vi "RT oscilloscope.vi"() -> ()   [LabVIEW 2023]
uses:
  <resource>/objmgr/ni.dex.rc
  <vilib>/rvi/interface/nirviReadWriteControl/nirviReadWriteControl.xnode
  <vilib>/rvi/interface/Simulation/niFpgaSimulationCallBeginRW.vi
  <vilib>/rvi/errors/niLvFpgaAdjustHostInterfaceError.vi
  <vilib>/rvi/interface/nirviMethod/nirviMethod.xnode
  <vilib>/FPGAPlugInAG/Dynamic/niLvFpga_Run_Dynamic.vi
  <vilib>/FPGAPlugInAG/Dynamic/niLvFpga_Reset_Dynamic.vi
  <vilib>/rvi/interface/nirviMethod/StockFPGA_InlinedMethodWaitForSingleIRQ.vi
  <vilib>/FPGAPlugInAG/Dynamic/niLvFpga_WaitOnIrq_Dynamic.vi
  <vilib>/FPGAPlugInAG/Dynamic/niLvFpga_AcknowledgeIrq_Dynamic.vi
  <vilib>/FPGAPlugInAG/Dynamic/niLvFpga_ReadFifo_Dynamic.vi
  <vilib>/rvi/errors/niLvFpgaMergeErrorWithErrorCode.vi
  <vilib>/rvi/interface/nirviOpenFPGA/nirviOpenFPGA.xnode
  <vilib>/rvi/interface/nirviCloseFPGA/nirviCloseFPGA.xnode
  <vilib>/FPGAPlugInAG/Dynamic/niLvFpga_Close_Dynamic.vi
  FPGA Bitfiles/Mainproject_FPGATarget_Icreadoutclocked_PcJtOPDfEmI.lvbitx
  Ic readout_clocked_delayed trigger_dist V3.vi
  Transport measurement/FPGA Bitfiles/transportmain_FPGATarget_oscilloscope_quBCWYi9ZeU.lvbitx
  oscilloscope.vi
  <vilib>/FPGAPlugInAG/cRIO-9063/niLvFpga_Open_cRIO-9063.vi
  <vilib>/rvi/interface/common/dynamic/niFpgaDynamicAddResources.vi
  <vilib>/LabVIEW Targets/FPGA/cRIO/shared/nicrio_ModuleControls/nicrio_cRIO-9775_RecordDataRates4ChansRing.ctl
  RT fast data.ctl
panel:
  out "VI Stop":bool
  out "error out 2":errorcluster
  out "error out":errorcluster
  in  "Parameters":T1={"Records Num"=10000, "AI Trigger Configuration"={"Trigger Slope"=enum."Positive", "Trigger Level"=0.1298828125, "Hystesis Value"=0.0, "AI Channel"=0}, "Record PreTrigger Samples"=1, "Record Samples"=16, "Ic Cut off or curve"=TRUE, "Gate wait time us"=150, "Record Data Rate"=1, "Count us half of T"=15, "Wait before trigger us"=10100, "Cutoff delay usec"=0} {"Record Data Rate" items=["20.000 MS/s (NI 9775)"=1, "10.00 MS/s (NI 9775)"=2, "6.667 MS/s (NI 9775)"=3, "5.000 MS/s (NI 9775)"=4, "2.500 MS/s (NI 9775)"=8, "1.667 MS/s (NI 9775)"=12, "1.250 MS/s (NI 9775)"=16, "1.000 MS/s (NI 9775)"=20, "833.333 KS/s (NI 9775)"=24, "714.286 KS/s (NI 9775)"=28, "625.000 KS/s (NI 9775)"=32, "555.556 KS/s (NI 9775)"=36, "500.000 KS/s (NI 9775)"=40, "454.545 KS/s (NI 9775)"=44, "416.667 KS/s (NI 9775)"=48, "384.615 KS/s (NI 9775)"=52, "357.143 KS/s (NI 9775)"=56, "333.333 KS/s (NI 9775)"=60, "312.500 KS/s (NI 9775)"=64, "294.118 KS/s (NI 9775)"=68, "277.778 KS/s (NI 9775)"=72, "263.158 KS/s (NI 9775)"=76, "250.000 KS/s (NI 9775)"=80, "238.095 KS/s (NI 9775)"=84, "227.273 KS/s (NI 9775)"=88, "217.391 KS/s (NI 9775)"=92, "208.333 KS/s (NI 9775)"=96, "200.000 KS/s (NI 9775)"=100, "192.308 KS/s (NI 9775)"=104, "185.185 KS/s (NI 9775)"=108, "178.571 KS/s (NI 9775)"=112, "172.414 KS/s (NI 9775)"=116, "166.667 KS/s (NI 9775)"=120, "161.290 KS/s (NI 9775)"=124, "156.250 KS/s (NI 9775)"=128, "151.515 KS/s (NI 9775)"=132, "147.059 KS/s (NI 9775)"=136, "142.857 KS/s (NI 9775)"=140, "138.889 KS/s (NI 9775)"=144, "135.135 KS/s (NI 9775)"=148, "131.579 KS/s (NI 9775)"=152, "128.205 KS/s (NI 9775)"=156, "125.000 KS/s (NI 9775)"=160, "121.951 KS/s (NI 9775)"=164, "119.048 KS/s (NI 9775)"=168, "116.279 KS/s (NI 9775)"=172, "113.636 KS/s (NI 9775)"=176, "111.111 KS/s (NI 9775)"=180, "108.696 KS/s (NI 9775)"=184, "106.383 KS/s (NI 9775)"=188, "104.167 KS/s (NI 9775)"=192, "102.041 KS/s (NI 9775)"=196, "100.000 KS/s (NI 9775)"=200, "50.000 KS/s (NI 9775)"=400, "33.333 KS/s (NI 9775)"=600, "25.000 KS/s (NI 9775)"=800, "20.000 KS/s (NI 9775)"=1000, "16.667 KS/s (NI 9775)"=1200, "14.286 KS/s (NI 9775)"=1400, "12.500 KS/s (NI 9775)"=1600, "11.111 KS/s (NI 9775)"=1800, "10.000 KS/s (NI 9775)"=2000, "9.091 KS/s (NI 9775)"=2200, "8.333 KS/s (NI 9775)"=2400, "7.692 KS/s (NI 9775)"=2600, "7.143 KS/s (NI 9775)"=2800, "6.667 KS/s (NI 9775)"=3000, "6.250 KS/s (NI 9775)"=3200, "5.882 KS/s (NI 9775)"=3400, "5.556 KS/s (NI 9775)"=3600, "5.000 KS/s (NI 9775)"=4000, "4.762 KS/s (NI 9775)"=4200, "4.545 KS/s (NI 9775)"=4400, "4.348 KS/s (NI 9775)"=4600, "4.167 KS/s (NI 9775)"=4800, "4.000 KS/s (NI 9775)"=5000, "3.846 KS/s (NI 9775)"=5200, "3.571 KS/s (NI 9775)"=5600, "3.333 KS/s (NI 9775)"=6000, "3.125 KS/s (NI 9775)"=6400, "2.941 KS/s (NI 9775)"=6800, "2.778 KS/s (NI 9775)"=7200, "2.632 KS/s (NI 9775)"=7600, "2.500 KS/s (NI 9775)"=8000, "2.381 KS/s (NI 9775)"=8400, "2.273 KS/s (NI 9775)"=8800, "2.174 KS/s (NI 9775)"=9200, "2.083 KS/s (NI 9775)"=9600, "2.000 KS/s (NI 9775)"=10000, "1.923 KS/s (NI 9775)"=10400, "1.852 KS/s (NI 9775)"=10800, "1.786 KS/s (NI 9775)"=11200, "1.724 KS/s (NI 9775)"=11600, "1.667 KS/s (NI 9775)"=12000, "1.613 KS/s (NI 9775)"=12400, "1.563 KS/s (NI 9775)"=12800, "1.515 KS/s (NI 9775)"=13200, "1.471 KS/s (NI 9775)"=13600, "1.429 KS/s (NI 9775)"=14000, "1.389 KS/s (NI 9775)"=14400, "1.351 KS/s (NI 9775)"=14800, "1.316 KS/s (NI 9775)"=15200, "1.282 KS/s (NI 9775)"=15600, "1.250 KS/s (NI 9775)"=16000, "1.220 KS/s (NI 9775)"=16400, "1.190 KS/s (NI 9775)"=16800, "1.163 KS/s (NI 9775)"=17200, "1.136 KS/s (NI 9775)"=17600, "1.111 KS/s (NI 9775)"=18000, "1.087 KS/s (NI 9775)"=18400, "1.064 KS/s (NI 9775)"=18800, "1.042 KS/s (NI 9775)"=19200, "1.020 KS/s (NI 9775)"=19600, "1.000 KS/s (NI 9775)"=20000, "0.980 KS/s (NI 9775)"=20400, "0.962 KS/s (NI 9775)"=20800, "0.943 KS/s (NI 9775)"=21200, "0.926 KS/s (NI 9775)"=21600, "0.909 KS/s (NI 9775)"=22000, "0.893 KS/s (NI 9775)"=22400, "0.877 KS/s (NI 9775)"=22800, "0.862 KS/s (NI 9775)"=23200, "0.847 KS/s (NI 9775)"=23600, "0.833 KS/s (NI 9775)"=24000, "0.820 KS/s (NI 9775)"=24400, "0.806 KS/s (NI 9775)"=24800, "0.794 KS/s (NI 9775)"=25200, "0.781 KS/s (NI 9775)"=25600, "0.694 KS/s (NI 9775)"=28800, "0.625 KS/s (NI 9775)"=32000, "0.568 KS/s (NI 9775)"=35200, "0.521 KS/s (NI 9775)"=38400, "0.446 KS/s (NI 9775)"=44800, "0.391 KS/s (NI 9775)"=51200, "0.347 KS/s (NI 9775)"=57600, "0.313 KS/s (NI 9775)"=64000]}
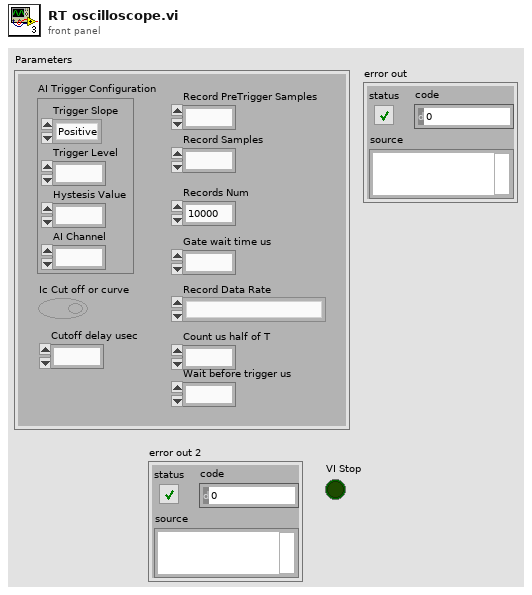
[diagram p1: front panel]
types:
  T1 = typedef "RT fast data.ctl" = cluster{"Records Num":i32, "AI Trigger Configuration":cluster{"Trigger Slope":enum8{"Positive", "Negative"}, "Trigger Level":fxp<+/-,17,5>, "Hystesis Value":fxp<+,16,4>, "AI Channel":u8}, "Record PreTrigger Samples":u32, "Record Samples":u32, "Ic Cut off or curve":bool, "Gate wait time us":u32, "Record Data Rate":T2, "Count us half of T":u32, "Wait before trigger us":u32, "Cutoff delay usec":u32}
  T2 = typedef "nicrio_cRIO-9775_RecordDataRates4ChansRing.ctl" = u16
  T3 = cluster{"Command":string, "Voltage":dbl, "Channel":string}
  T4 = cluster{"Trigger Slope":enum8{"Positive", "Negative"}, "Trigger Level":fxp<+/-,17,5>, "Hystesis Value":fxp<+,16,4>, "AI Channel":u8}
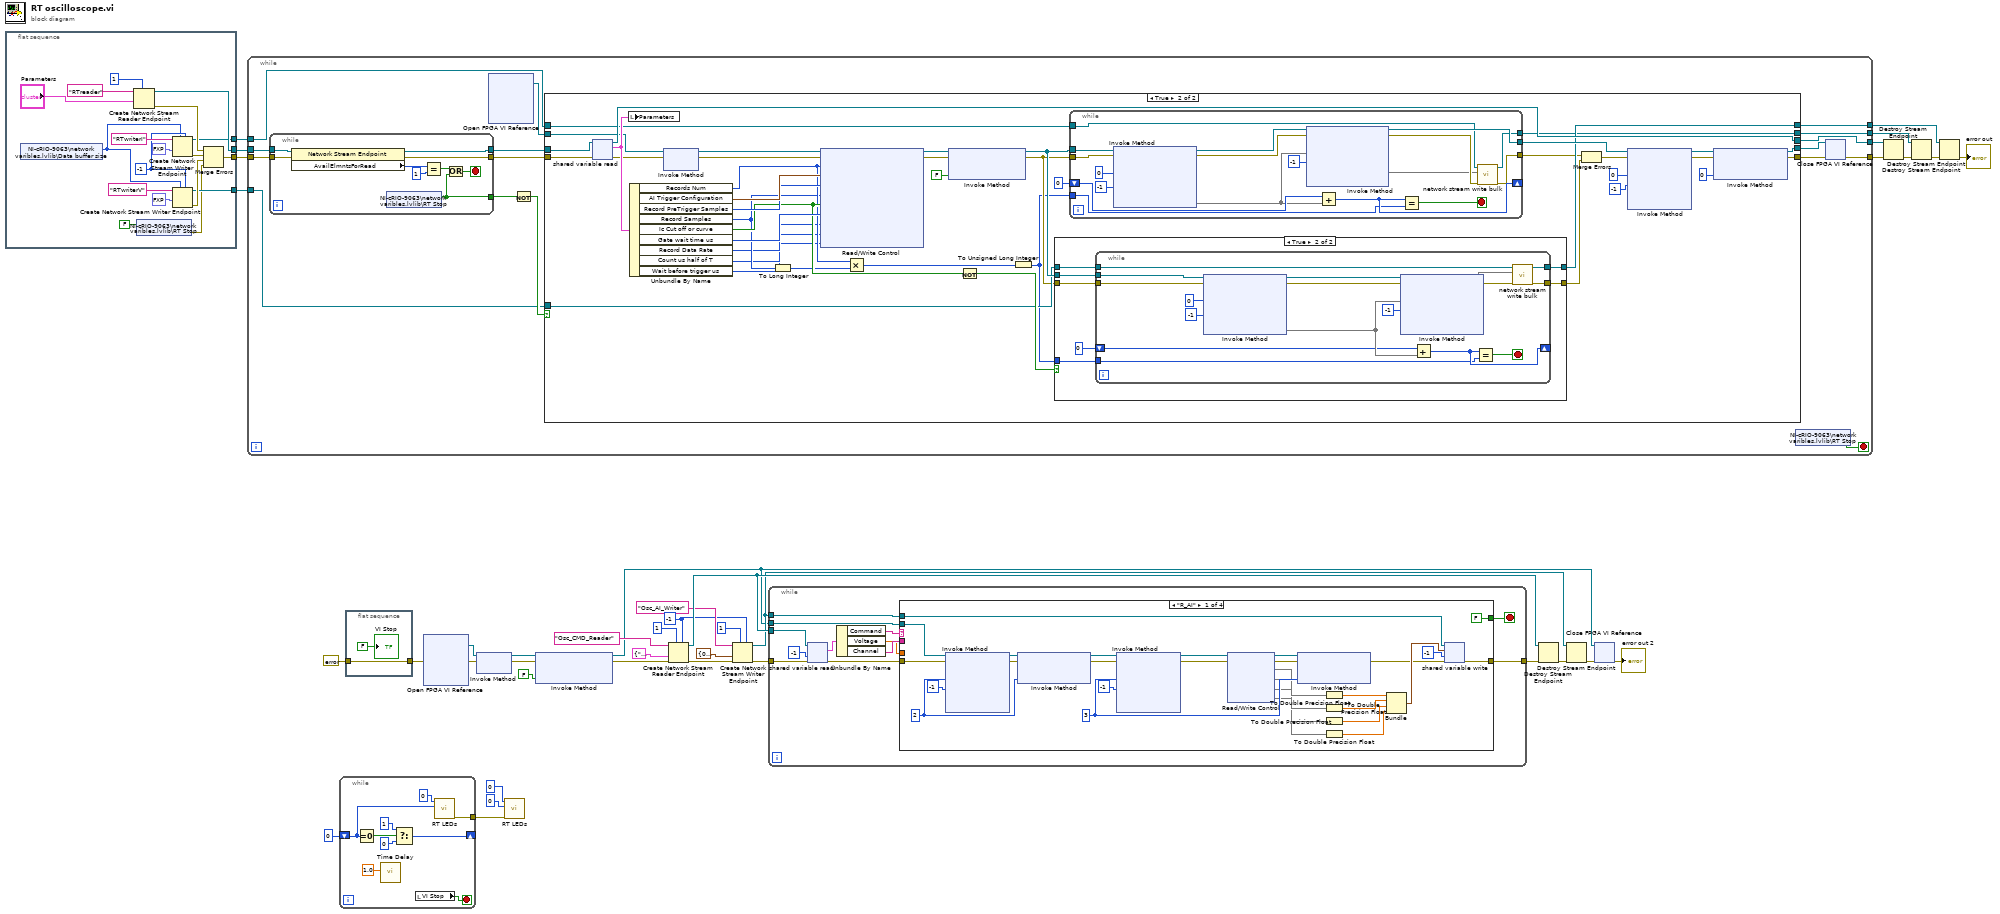
[diagram p0: block diagram]
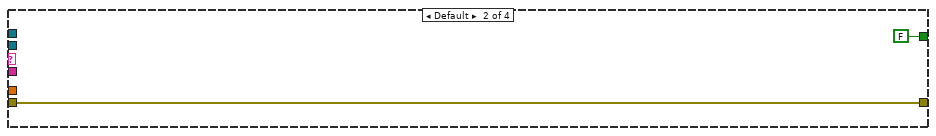
[diagram p2: hidden frame]
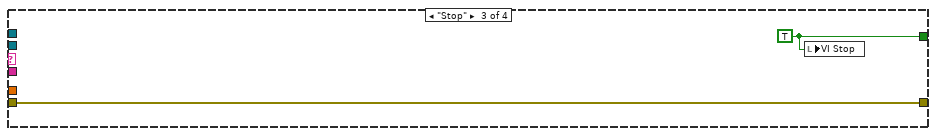
[diagram p3: hidden frame]
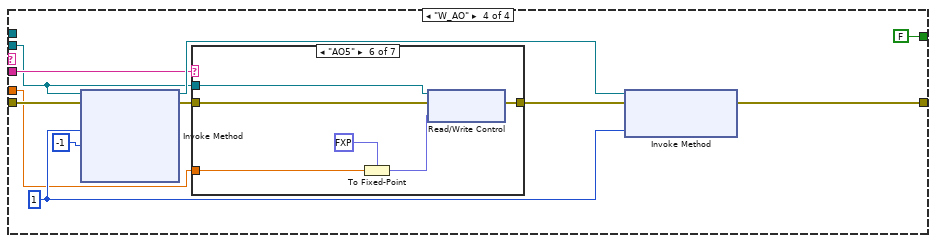
[diagram p4: hidden frame]
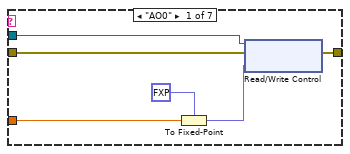
[diagram p5: hidden frame]
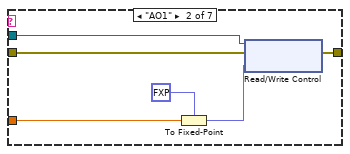
[diagram p6: hidden frame]
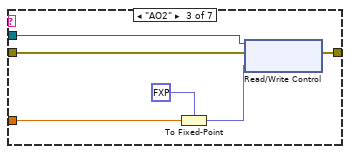
[diagram p7: hidden frame]
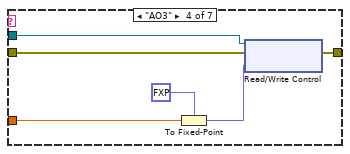
[diagram p8: hidden frame]
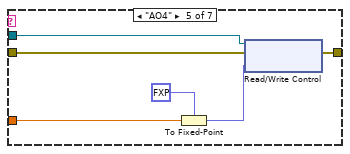
[diagram p9: hidden frame]
diagram:
  w1 = -1 ("timeout in ms (-1)")
  n1 = flat-sequence {
    tunnel: [w55] -> w39
    tunnel: [w45] -> w38
    tunnel: [w44] -> w33
    tunnel: [w43] -> w32
    frame #0 {
      w50 = -1 ("timeout in ms (-1)")
      n2 = shared-variable "NI-cRIO-9063\\network varibles.lvlib\\Data buffer size"() -> (w49:i32)  [unwired: 1 in, 1 out]
      n3 = Create Network Stream Reader Endpoint(7:1 ("reader buffer size"), 9:"Parameters", 11:"RTreader" ("reader name")) -> (0:w48:errorcluster, 3:w55:refnum<k21>)  [unwired: 4 in]
      n4 = shared-variable "NI-cRIO-9063\\network varibles.lvlib\\RT Stop"(FALSE ("RT Stop")) -> (error out=w41:errorcluster)  [unwired: 1 in]
      n5 = Create Network Stream Writer Endpoint(5:w50, 7:w49, 9:fxp<+/-,17,5> 0.0, 11:"RTwriterI" ("writer name")) -> (0:w47:errorcluster, 3:w44:refnum<k21>)  [unwired: 3 in]
      n6 = Create Network Stream Writer Endpoint(5:w50, 7:w49, 9:fxp<+/-,17,5> 0.0, 11:"RTwriterV" ("writer name")) -> (0:w46:errorcluster, 3:w43:refnum<k21>)  [unwired: 3 in]
      n7 = Merge Errors(w48, w47, w46, w41) -> (w45:errorcluster)
    }
  }
  n8 = while {
    tunnel: w39 -> [w73]
    tunnel: w38 -> [w72]
    tunnel: [w59] -> w29
    tunnel: [w69] -> w37
    tunnel: w33 -> [w65]
    tunnel: w32 -> [w64]
    tunnel: [w63] -> w31
    tunnel: [w62] -> w30
    stop <- w68 stop-if-true
    n9 = while {
      tunnel: w73 -> [w173]
      tunnel: w72 -> [w172]
      tunnel: [w171] -> w71
      tunnel: [w170] -> w70
      tunnel: [w165] -> w58
      stop <- w166 stop-if-true
      n10 = property class="Network Stream Endpoint"(reference=w173, error in=w172) -> (reference out=w171:refnum<k21>, error out=w170:errorcluster, "AvailElmntsForRead"=w169:i32)
      n11 = shared-variable "NI-cRIO-9063\\network varibles.lvlib\\RT Stop"() -> (w165:bool)  [unwired: 1 in, 1 out]
      n12 = Equal?(x=w169, y=1) -> (x = y?=w167:bool)
      n13 = Or(x=w167, y=w165) -> (x .or. y?=w166:bool)
    }
    n14 = xnode "Open FPGA VI Reference"() -> ("FPGA VI Reference Out"=w66:refnum<k20>)  [unwired: 2 in, 1 out]
    n15 = Not(x=w58) -> (.not. x?=w67:bool)
    n16 = case shown="True" w67 {
      tunnel: w71 -> [w77 w115]
      tunnel: w70 -> [w78 w114]
      tunnel: [w76 w105] -> w61
      tunnel: [w78 w104] -> w60
      tunnel: [w77 w103] -> w69
      tunnel: w66 -> [w76 w96]
      tunnel: w65 -> [w75 w88]
      tunnel: w64 -> [w74 w90]
      tunnel: [w75 w87] -> w63
      tunnel: [w74 w89] -> w62
      frame False {
      }
      frame True {
        n17 = shared-variable-read(w115, w114) -> (w103:refnum<k21>, w95:errorcluster, w113:T1)  [unwired: 1 in, 1 out]
        n18 = local write "Parameters"(w113) -> ()
        n19 = Unbundle By Name(w113) -> ("Records Num"=w94:i32, "AI Trigger Configuration"=w117:T4, "Record PreTrigger Samples"=w116:u32, "Record Samples"=w93:u32, "Ic Cut off or curve"=w99:bool, "Gate wait time us"=w112:u32, "Record Data Rate"=w85:T2, "Count us half of T"=w80:u32, "Wait before trigger us"=w79:u32)
        n20 = xnode "Invoke Method"("FPGA VI Reference In"=w96, "error in"=w95) -> ("FPGA VI Reference Out"=w119:refnum<k20>, "error out"=w97:errorcluster)
        n21 = To Long Integer(number=w93) -> (32bit integer=w92:i32)
        n22 = xnode "Read/Write Control"("FPGA VI Reference In"=w119, "error in"=w97, "Records Num"=w94, "AI Trigger Configuration"=w117, "Record PreTrigger Samples"=w116, "Record Samples"=w93, "Ic Cut off or curve"=w99, "Gate wait time us"=w112, "Record Data Rate"=w85, "Count ms"=w80, "Wait before trigger us"=w79) -> ("FPGA VI Reference Out"=w120:refnum<k20>, "error out"=w81:errorcluster)
        n23 = Multiply(x=w94, y=w92) -> (x*y=w91:i32)
        n24 = xnode "Invoke Method"("FPGA VI Reference In"=w120, "error in"=w81, "Wait Until Done (F)"=FALSE) -> ("FPGA VI Reference Out"=w102:refnum<k20>, "error out"=w83:errorcluster)
        n25 = Not(x=w99) -> (.not. x?=w98:bool)
        n26 = To Unsigned Long Integer(number=w91) -> (unsigned 32bit integer=w82:u32)
        n27 = case shown="True" w98 {
          tunnel: w102 -> [_ w147]
          tunnel: [w139 w141] -> w101
          tunnel: w90 -> [w140 w146]
          tunnel: [w140 w142] -> w89
          tunnel: w83 -> [w139 w144]
          tunnel: w82 -> [_ w143]
          frame False {
          }
          frame True {
            n28 = while {
              tunnel: w147 -> [w157]
              tunnel: w146 -> [w152]
              shift-right: [w154] -> _
              shift-left: u32 0 ("Number of Elements") -> [w156]
              tunnel: w144 -> [w155]
              tunnel: w143 -> [w153]
              tunnel: [w151] -> w142
              tunnel: [w148] -> w141
              stop <- w158 stop-if-true
              n29 = xnode "Invoke Method"("FPGA VI Reference In"=w157, "error in"=w155, "Number of Elements"=u32 0, "Timeout (ms)"=-1) -> ("FPGA VI Reference Out"=w162:refnum<k20>, "error out"=w163:errorcluster, "Elements Remaining"=w164)  [unwired: 1 out]
              n30 = xnode "Invoke Method"("FPGA VI Reference In"=w162, "error in"=w163, "Number of Elements"=w164, "Timeout (ms)"=-1) -> ("error out"=w149:errorcluster, "Data"=w150:void[])  [unwired: 2 out]
              n31 = Add(x=w156, y=w164) -> (x+y=w154:u32)
              n32 = Equal?(x=w154, y=w153) -> (x = y?=w158:bool)
              n33 = call "network stream write bulk.vi"("error in (no error)"=w149, "Data"=w150, "endpoint in"=w152) -> ("error out"=w148:errorcluster, "endpoint out"=w151:refnum<k21>)  [unwired: 7 in]
            }
          }
        }
        n34 = while {
          tunnel: w88 -> [w122]
          tunnel: [w123] -> w87
          tunnel: w102 -> [w136]
          tunnel: [w137] -> w111
          tunnel: w83 -> [w134]
          tunnel: [w124] -> w86
          shift-right: [w128] -> _
          shift-left: u32 0 ("Number of Elements") -> [w130]
          tunnel: w82 -> [w127]
          stop <- w126 stop-if-true
          n35 = xnode "Invoke Method"("FPGA VI Reference In"=w136, "error in"=w134, "Number of Elements"=u32 0, "Timeout (ms)"=-1) -> ("FPGA VI Reference Out"=w135:refnum<k20>, "error out"=w133:errorcluster, "Elements Remaining"=w129)  [unwired: 1 out]
          n36 = xnode "Invoke Method"("FPGA VI Reference In"=w135, "error in"=w133, "Number of Elements"=w129, "Timeout (ms)"=-1) -> ("FPGA VI Reference Out"=w137:refnum<k20>, "error out"=w125:errorcluster, "Data"=w121:void[])  [unwired: 1 out]
          n37 = Add(x=w130, y=w129) -> (x+y=w128:u32)
          n38 = Equal?(x=w128, y=w127) -> (x = y?=w126:bool)
          n39 = call "network stream write bulk.vi"("error in (no error)"=w125, "Data"=w121, "endpoint in"=w122) -> ("error out"=w124:errorcluster, "endpoint out"=w123:refnum<k21>)  [unwired: 7 in]
        }
        n40 = Merge Errors(w86, w101) -> (w100:errorcluster)
        n41 = xnode "Invoke Method"("FPGA VI Reference In"=w111, "error in"=w100, "IRQ Number(s)"=0, "Timeout (ms)"=-1) -> ("FPGA VI Reference Out"=w108:refnum<k20>, "error out"=w107:errorcluster)  [unwired: 2 out]
        n42 = xnode "Invoke Method"("FPGA VI Reference In"=w108, "error in"=w107, "IRQ Number(s)"=0) -> ("FPGA VI Reference Out"=w105:refnum<k20>, "error out"=w104:errorcluster)
      }
    }
    n43 = shared-variable "NI-cRIO-9063\\network varibles.lvlib\\RT Stop"() -> (w68:bool)  [unwired: 1 in, 1 out]
    n44 = xnode "Close FPGA VI Reference"("FPGA VI Reference In"=w61, "error in"=w60) -> ("error out"=w59:errorcluster)
  }
  n45 = while {
    shift-right: [w177] -> _
    shift-left: 0 ("State") -> [w181]
    tunnel: [w174] -> w4
    stop <- w175 stop-if-true
    n46 = Equal To 0?(x=w181) -> (x = 0?=w180:bool)
    n47 = call "Time Delay"("Delay Time (s)"=1.0) -> ()  [unwired: 10 in, 1 out]
    n48 = Select(t=1, s=w180, f=0) -> (s? t:f=w177:i32)
    n49 = local read "VI Stop"() -> (w175:bool)
    n50 = call <vilib>:"RT LEDs.vi"("State"=w181, "LED Num"=0) -> ("error out"=w174:errorcluster)  [unwired: 4 in, 1 out]
  }
  n51 = flat-sequence {
    tunnel: errorcluster {"status"=FALSE, "code"=0, "source"=""} ("error in (no error)") -> [w184]
    tunnel: [w184] -> w2
    frame #0 {
      "VI Stop" <- FALSE ("VI Stop")
    }
  }
  n52 = xnode "Open FPGA VI Reference"("error in"=w2) -> ("FPGA VI Reference Out"=w24:refnum<k20>, "error out"=w23:errorcluster)  [unwired: 1 in]
  n53 = xnode "Invoke Method"("FPGA VI Reference In"=w24, "error in"=w23) -> ("FPGA VI Reference Out"=w25:refnum<k20>, "error out"=w22:errorcluster)
  n54 = call <vilib>:"RT LEDs.vi"("error in (no error)"=w4, "State"=0, "LED Num"=0) -> ()  [unwired: 3 in, 2 out]
  n55 = xnode "Invoke Method"("FPGA VI Reference In"=w25, "error in"=w22, "Wait Until Done (F)"=FALSE) -> ("FPGA VI Reference Out"=w11:refnum<k20>, "error out"=w17:errorcluster)
  n56 = Create Network Stream Reader Endpoint(5:w1, 7:1 ("reader buffer size"), 8:w17, 9:T3 {"Command"="", "Voltage"=0.0, "Channel"=""} ("Write cluster"), 11:"Osc_CMD_Reader" ("reader name")) -> (0:w14:errorcluster, 3:w20:refnum<k21>)  [unwired: 2 in]
  n57 = Create Network Stream Writer Endpoint(5:w1, 7:1 ("writer buffer size"), 8:w14, 9:cluster{dbl, dbl, dbl, dbl} {0.0, 0.0, 0.0, 0.0} ("output cluster"), 11:"Osc_AI_Writer" ("reader name")) -> (0:w9:errorcluster, 3:w13:refnum<k21>)  [unwired: 2 in]
  n58 = while {
    tunnel: w9 -> [w196]
    tunnel: w20 -> [w195]
    tunnel: w11 -> [w191]
    tunnel: [w186] -> w21
    tunnel: w13 -> [w187]
    stop <- w185 stop-if-true
    n59 = shared-variable-read(w195, w196, -1 ("timeout ms (-1)")) -> (w190:errorcluster, w193:T3)  [unwired: 2 out]
    n60 = Unbundle By Name(w193) -> ("Command"=w192:string, "Voltage"=w188:dbl, "Channel"=w189:string)
    n61 = case shown="\"R_AI\"" w192 {
      tunnel: w191 -> [w219 _ _ w232]
      tunnel: w190 -> [w220 w225 w228 w235]
      tunnel: w189 -> [_ _ _ w233]
      tunnel: w188 -> [_ _ _ w231]
      tunnel: [w198 w225 w228 w230] -> w186
      tunnel: w187 -> [w210 _ _ _]
      tunnel: [FALSE FALSE w227 FALSE] -> w185
      frame "R_AI" {
        w218 = 3 ("IRQ Number(s)")
        w222 = 2 ("IRQ Number(s)")
        n62 = xnode "Invoke Method"("FPGA VI Reference In"=w219, "error in"=w220, "IRQ Number(s)"=w222, "Timeout (ms)"=-1) -> ("FPGA VI Reference Out"=w223:refnum<k20>, "error out"=w224:errorcluster)  [unwired: 2 out]
        n63 = xnode "Invoke Method"("FPGA VI Reference In"=w223, "error in"=w224, "IRQ Number(s)"=w222) -> ("FPGA VI Reference Out"=w216:refnum<k20>, "error out"=w215:errorcluster)
        n64 = xnode "Invoke Method"("FPGA VI Reference In"=w216, "error in"=w215, "IRQ Number(s)"=w218, "Timeout (ms)"=-1) -> ("FPGA VI Reference Out"=w214:refnum<k20>, "error out"=w213:errorcluster)  [unwired: 2 out]
        n65 = xnode "Read/Write Control"("FPGA VI Reference In"=w214, "error in"=w213) -> ("FPGA VI Reference Out"=w212:refnum<k20>, "error out"=w211:errorcluster, "Mod1/AI0"=w209, "Mod1/AI1"=w208, "Mod1/AI2"=w207, "Mod1/AI3"=w206)
        n66 = xnode "Invoke Method"("FPGA VI Reference In"=w212, "error in"=w211, "IRQ Number(s)"=w218) -> ("error out"=w200:errorcluster)  [unwired: 1 out]
        n67 = To Double Precision Float(number=w209) -> (double precision float=w205:dbl)
        n68 = To Double Precision Float(number=w208) -> (double precision float=w204:dbl)
        n69 = To Double Precision Float(number=w207) -> (double precision float=w203:dbl)
        n70 = To Double Precision Float(number=w206) -> (double precision float=w202:dbl)
        n71 = Bundle(w205, w204, w203, w202) -> (w201:cluster{dbl, dbl, dbl, dbl})  [unwired: 1 in]
        n72 = shared-variable-write(w210, w200, w201, -1 ("timeout ms (-1)")) -> (w198:errorcluster)  [unwired: 2 out]
      }
      frame Default {
      }
      frame "Stop" {
        w227 = TRUE
        n73 = local write "VI Stop"(w227) -> ()
      }
      frame "W_AO" {
        w236 = 1 ("IRQ Number(s)")
        n74 = xnode "Invoke Method"("FPGA VI Reference In"=w232, "error in"=w235, "IRQ Number(s)"=w236, "Timeout (ms)"=-1) -> ("FPGA VI Reference Out"=w237:refnum<k20>, "error out"=w238:errorcluster)  [unwired: 2 out]
        n75 = case shown="\"AO5\"" w233 {
          tunnel: w232 -> [w245 w249 w255 w261 w267 w273 _]
          tunnel: w231 -> [w242 w247 w254 w260 w265 w271 _]
          tunnel: w238 -> [w241 w248 w253 w259 w266 w272 w276]
          tunnel: [w240 w246 w252 w258 w264 w270 w276] -> w239
          frame "AO0" {
            n76 = To Fixed-Point(fixed-point type=fxp<+/-,20,5> 0.0 ("Mod3/AO0"), number=w242) -> (fixed-point=w243:fxp<+/-,20,5>)
            n77 = xnode "Read/Write Control"("FPGA VI Reference In"=w245, "error in"=w241, "Mod3/AO0"=w243) -> ("error out"=w240:errorcluster)  [unwired: 1 out]
          }
          frame "AO1" {
            n78 = To Fixed-Point(fixed-point type=fxp<+/-,20,5> 0.0 ("Mod3/AO0"), number=w247) -> (fixed-point=w250:fxp<+/-,20,5>)
            n79 = xnode "Read/Write Control"("FPGA VI Reference In"=w249, "error in"=w248, "Mod3/AO1"=w250) -> ("error out"=w246:errorcluster)  [unwired: 1 out]
          }
          frame "AO2" {
            n80 = To Fixed-Point(fixed-point type=fxp<+/-,20,5> 0.0 ("Mod3/AO0"), number=w254) -> (fixed-point=w256:fxp<+/-,20,5>)
            n81 = xnode "Read/Write Control"("FPGA VI Reference In"=w255, "error in"=w253, "Mod3/AO2"=w256) -> ("error out"=w252:errorcluster)  [unwired: 1 out]
          }
          frame "AO3" {
            n82 = To Fixed-Point(fixed-point type=fxp<+/-,20,5> 0.0 ("Mod3/AO0"), number=w260) -> (fixed-point=w262:fxp<+/-,20,5>)
            n83 = xnode "Read/Write Control"("FPGA VI Reference In"=w261, "error in"=w259, "Mod3/AO3"=w262) -> ("error out"=w258:errorcluster)  [unwired: 1 out]
          }
          frame "AO4" {
            n84 = To Fixed-Point(fixed-point type=fxp<+/-,20,5> 0.0 ("Mod3/AO0"), number=w265) -> (fixed-point=w268:fxp<+/-,20,5>)
            n85 = xnode "Read/Write Control"("FPGA VI Reference In"=w267, "error in"=w266, "Mod3/AO4"=w268) -> ("error out"=w264:errorcluster)  [unwired: 1 out]
          }
          frame "AO5" {
            n86 = To Fixed-Point(fixed-point type=fxp<+/-,20,5> 0.0 ("Mod3/AO0"), number=w271) -> (fixed-point=w274:fxp<+/-,20,5>)
            n87 = xnode "Read/Write Control"("FPGA VI Reference In"=w273, "error in"=w272, "Mod3/AO5"=w274) -> ("error out"=w270:errorcluster)  [unwired: 1 out]
          }
          frame Default {
          }
        }
        n88 = xnode "Invoke Method"("FPGA VI Reference In"=w237, "error in"=w239, "IRQ Number(s)"=w236) -> ("error out"=w230:errorcluster)  [unwired: 1 out]
      }
    }
  }
  n89 = Destroy Stream Endpoint(8:w21, 11:w20) -> (0:w19:errorcluster)
  n90 = Destroy Stream Endpoint(8:w19, 11:w13) -> (0:w10:errorcluster)
  n91 = xnode "Close FPGA VI Reference"("FPGA VI Reference In"=w11, "error in"=w10) -> ("error out"=→"error out 2":errorcluster)
  n92 = Destroy Stream Endpoint(8:w29, 11:w37) -> (0:w36:errorcluster)
  n93 = Destroy Stream Endpoint(8:w36, 11:w31) -> (0:w35:errorcluster)
  n94 = Destroy Stream Endpoint(8:w35, 11:w30) -> (0:→"error out":errorcluster)
